vi "XNETDB Add.vi"(8 "error in (no error)":errorcluster, 10 "DB Alias data":T1, 11 "Databases Section Ref":T2 format="%.0x") -> (0 "error out":errorcluster)   [LabVIEW 2018, in "CAN Gateway System Explorer.lvlib"]
uses:
  CAN Gateway System Explorer.lvlib
  <vilib>/NI Veristand/Custom Device API/Custom Device Item Ref.ctl
  Types/Alias DB data.ctl
  Shared/Constants.vi
  <vilib>/NI/NI VeriStand Advanced SysDef API/_SubVIs/SysDef.Property.Set.String.vi
  <vilib>/NI/NI VeriStand Advanced SysDef API/SysDef API/Advanced System Definition.lvlib
  Shared/CAN Gateway Shared.lvlib
  <vilib>/NI Veristand/Custom Device API/Custom Device API.lvlib
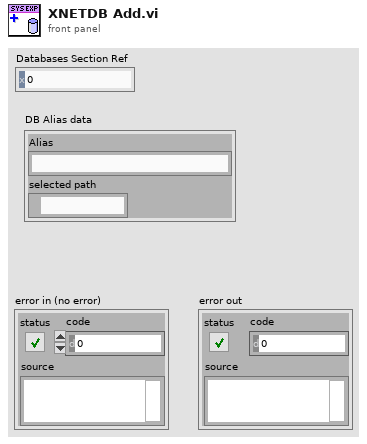
[diagram p1: front panel]
types:
  T1 = typedef "CAN Gateway System Explorer.lvlib/Alias DB data.ctl" = cluster{"Alias":string, "selected path":path}
  T2 = typedef "Custom Device API.lvlib/Custom Device Item Ref.ctl" = u64
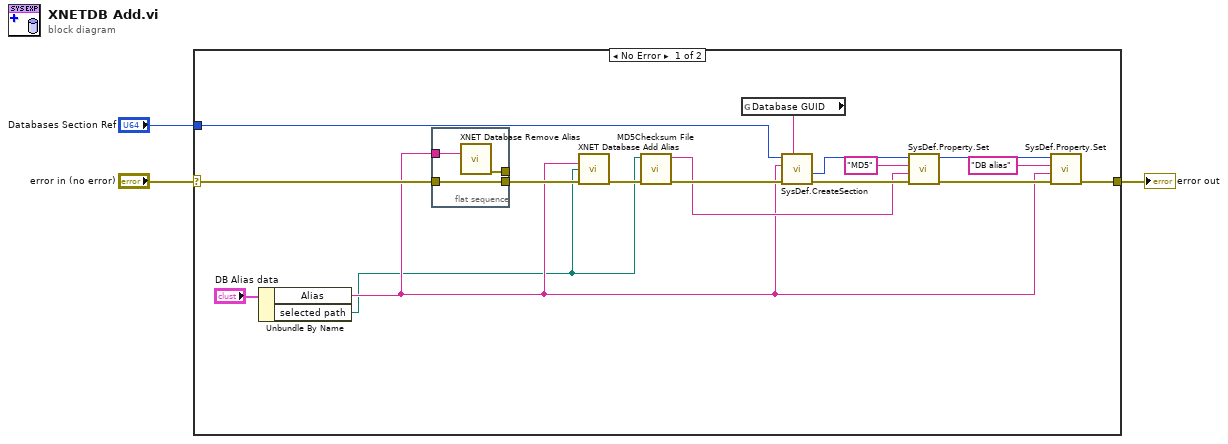
[diagram p0: block diagram]
diagram:
  n1 = case shown="No Error" "error in (no error)" {
    selector: "error in (no error)" -> [w18 w24]
    tunnel: "Databases Section Ref" -> [w20 _]
    tunnel: [w19 w24] -> w2
    frame No Error {
      n2 = Unbundle By Name("DB Alias data") -> ("Alias"=w6:string, "selected path"=w5:path)
      n3 = flat-sequence {
        tunnel: [w23] -> w8
        tunnel: w18 -> [w23]
        tunnel: [w22] -> _
        tunnel: w6 -> [w21]
        frame #0 {
          n4 = call <vilib>:"XNET Database Remove Alias.vi"("alias"=w21) -> ("error out"=w22:errorcluster)  [unwired: 14 in]
        }
      }
      n5 = call <vilib>:"XNET Database Add Alias.vi"("alias"=w6, "filepath"=w5, "error in (no error)"=w8) -> ("error out"=w17:errorcluster)  [unwired: 12 in]
      n6 = call <vilib>:"MD5Checksum File.vi"("error in (no error)"=w17, "Path"=w5) -> ("error out"=w10:errorcluster, "MD5 message-digest"=w9:string)  [unwired: 8 in]
      n7 = global read "Constants.vi" "Database GUID"() -> (w4:string)
      n8 = call <vilib>:"SysDef.CreateSection.vi"("GUID"=w4, "error in (no error)"=w10, "Name"=w6, "nodeID"=w20) -> ("error out"=w15:errorcluster, "New NodeID"=w16:u64)  [unwired: 4 in, 2 out]
      n9 = call-poly <vilib>:"SysDef.Property.Set.vi"("error in (no error)"=w15, "Value"=w9, "Property Name"="MD5", "nodeID"=w16) -> ("error out"=w14:errorcluster, "nodeID out"=w13:u64)  [unwired: 6 in]
      n10 = call-poly <vilib>:"SysDef.Property.Set.vi"("error in (no error)"=w14, "Value"=w6, "Property Name"="DB alias", "nodeID"=w13) -> ("error out"=w19:errorcluster)  [unwired: 6 in, 1 out]
    }
    frame Error {
    }
  }
  "error out" <- w2
